vi "Status Update.vi"(8 "error in (no error)":errorcluster, 10 "Status":string, 11 "Test in":refnum<class "Test.lvclass">) -> (0 "error out":errorcluster, 3 "Test out":refnum<class "Test.lvclass">)   [LabVIEW 2017, in "Test.lvlib" / "Test.lvclass"]
uses:
  Test.lvclass
  C:/Program Files (x86)/National Instruments/LabVIEW 2017/vi.lib/ActorFramework/Actor/Actor.lvclass
  <vilib>/ActorFramework/Actor/Actor.lvclass/Actor.ctl
  Test.lvclass/Test.ctl
  Test Messages/Send Status String Msg/Status String Msg.lvclass/Status String Msg.ctl
  <vilib>/ActorFramework/Message Enqueuer/Message Enqueuer.lvclass/Message Enqueuer.ctl
  <vilib>/ActorFramework/Message Enqueuer/Enqueue.vi
  Test Messages/Send Status String Msg/Status String Msg.lvclass
  C:/Program Files (x86)/National Instruments/LabVIEW 2017/vi.lib/ActorFramework/Message/Message.lvclass
  <vilib>/ActorFramework/Message Priority Queue/Priority Enqueue.vi
  <vilib>/ActorFramework/Actor/Actor.lvclass
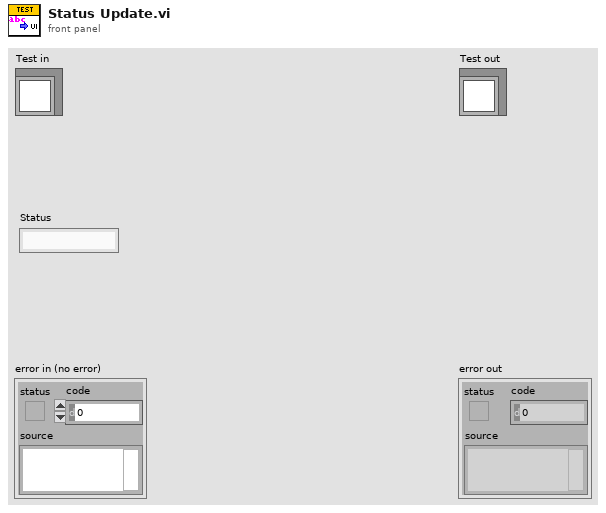
[diagram p1: front panel]
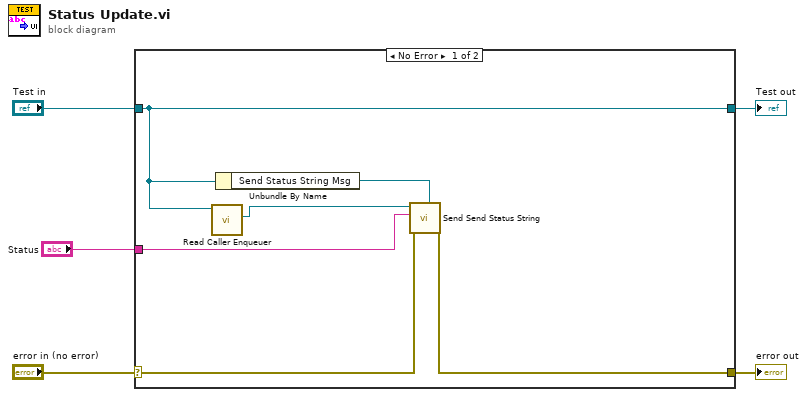
[diagram p0: block diagram]
diagram:
  n1 = case shown="No Error" "error in (no error)" {
    selector: "error in (no error)" -> [w7 w13]
    tunnel: [w6 w13] -> w4
    tunnel: [w10 w12] -> w2
    tunnel: "Test in" -> [w10 w12]
    tunnel: "Status" -> [w8 _]
    frame No Error {
      n2 = call <vilib>:"Read Caller Enqueuer.vi"("Actor"=w10) -> ("Caller Enqueuer"=w9:refnum<class "Message Enqueuer.lvclass">)  [unwired: 10 in]
      n3 = Unbundle By Name(w10) -> ("Send Status String Msg"=w11:refnum<class "Status String Msg.lvclass">)
      n4 = call "Send Send Status String.vi"("Message Type"=w11, "error in (no error)"=w7, "Status"=w8, "Message Enqueuer"=w9) -> ("error out"=w6:errorcluster)  [unwired: 6 in, 1 out]
    }
    frame Error {
    }
  }
  "error out" <- w4
  "Test out" <- w2
